vi "Equation.vi"(5 "Target height":dbl, 6 "Auto find":bool, 7 "Distance on ground (X)":dbl, 8 "RPM":dbl, 9 "zAvit":dbl) -> (0 "Risky!":bool, 1 "Calculated height":dbl, 2 "RPM":dbl, 3 "zAvit":dbl, 4 "Capable":bool)   [LabVIEW 2012]
panel:
  in  "K6":dbl
  in  "K5":dbl
  in  "K4":dbl
  in  "K3":dbl
  in  "K2":dbl
  in  "K1":dbl
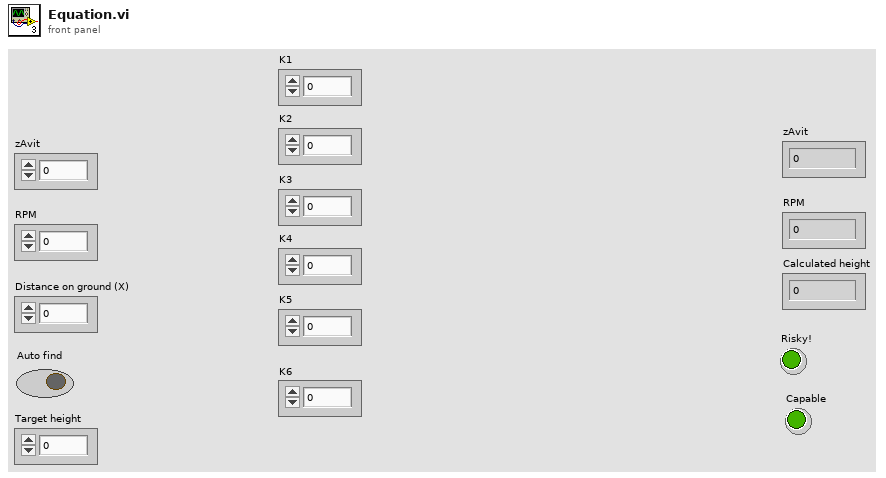
[diagram p1: front panel]
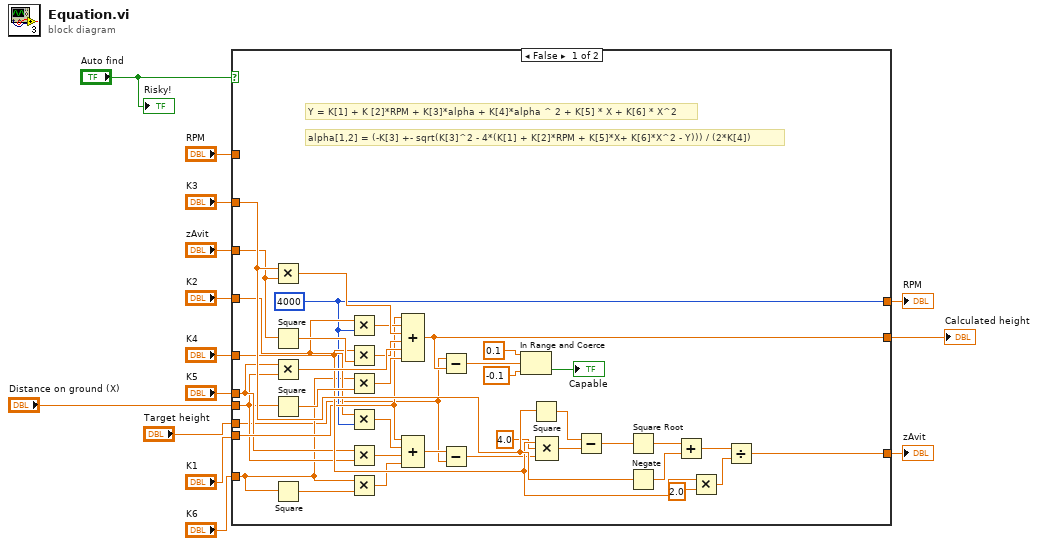
[diagram p0: block diagram]
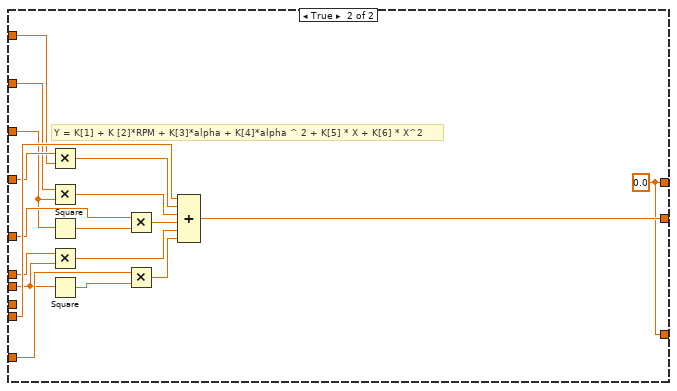
[diagram p2: hidden frame]
diagram:
  n1 = case shown="False" "Auto find" {
    tunnel: "K1" -> [w28 w65]
    tunnel: "K2" -> [w27 w64]
    tunnel: "RPM" -> [_ w63]
    tunnel: "K3" -> [w36 w62]
    tunnel: "K4" -> [w30 w61]
    tunnel: "zAvit" -> [w35 w56]
    tunnel: "K5" -> [w24 w59]
    tunnel: "K6" -> [w20 w58]
    tunnel: "Distance on ground (X)" -> [w23 w55]
    tunnel: [w26 w53] -> w4
    tunnel: [w33 w54] -> w3
    tunnel: [w47 w53] -> w2
    tunnel: "Target height" -> [w17 _]
    frame False {
      w26 = 4000
      # "alpha[1,2] = (-K[3] +- sqrt(K[3]^2 - 4*(K[1] + K[2]*RPM + K[5]*X+ K[6]*X^2 - Y))) / (2*K[4])"
      # "Y = K[1] + K [2]*RPM + K[3]*alpha + K[4]*alpha ^ 2 + K[5] * X + K[6] * X^2"
      n2 = Multiply(x=w36, y=w35) -> (x*y=w43:dbl)
      n3 = Square(x=w35) -> (x^2=w41:dbl)
      n4 = Multiply(x=w24, y=w23) -> (x*y=w45:dbl)
      n5 = Square(x=w23) -> (x^2=w34:dbl)
      n6 = Square(x=w20) -> (x^2=w21:dbl)
      n7 = Multiply(x=w27, y=w26) -> (x*y=w42:dbl)
      n8 = Multiply(x=w30, y=w41) -> (x*y=w44:dbl)
      n9 = Multiply(x=w20, y=w34) -> (x*y=w46:dbl)
      n10 = Multiply(x=w27, y=w26) -> (x*y=w25:dbl)
      n11 = Multiply(x=w24, y=w23) -> (x*y=w22:dbl)
      n12 = Multiply(x=w20, y=w21) -> (x*y=w18:dbl)
      n13 = Compound Arithmetic op=ADD(w28, w42, w43, w44, w45, w46) -> (w33:dbl)
      n14 = Compound Arithmetic op=ADD(w28, w25, w22, w18) -> (w19:dbl)
      n15 = Subtract(x=w17, y=w33) -> (x-y=w40:dbl)
      n16 = Subtract(x=w19, y=w17) -> (x-y=w16:dbl)
      n17 = In Range and Coerce(upper limit=0.1, x=w40, lower limit=-0.1) -> (In Range?=→"Capable":bool)  [unwired: 1 out]
      n18 = Square(x=w36) -> (x^2=w31:dbl)
      n19 = Compound Arithmetic op=MULTIPLY(w30, 4.0 ("y"), w16) -> (w15:dbl)
      n20 = Subtract(x=w31, y=w15) -> (x-y=w32:dbl)
      n21 = Square Root(x=w32) -> (sqrt(x)=w50:dbl)
      n22 = Negate(x=w36) -> (-x=w49:dbl)
      n23 = Add(x=w50, y=w49) -> (x+y=w48:dbl)
      n24 = Multiply(x=w30, y=2.0) -> (x*y=w51:dbl)
      n25 = Divide(x=w48, y=w51) -> (x/y=w47:dbl)
    }
    frame True {
      w53 = 0.0
      # "Y = K[1] + K [2]*RPM + K[3]*alpha + K[4]*alpha ^ 2 + K[5] * X + K[6] * X^2"
      n26 = Multiply(x=w64, y=w63) -> (x*y=w66:dbl)
      n27 = Multiply(x=w62, y=w56) -> (x*y=w67:dbl)
      n28 = Square(x=w56) -> (x^2=w60:dbl)
      n29 = Multiply(x=w59, y=w55) -> (x*y=w69:dbl)
      n30 = Square(x=w55) -> (x^2=w57:dbl)
      n31 = Multiply(x=w61, y=w60) -> (x*y=w68:dbl)
      n32 = Multiply(x=w58, y=w57) -> (x*y=w70:dbl)
      n33 = Compound Arithmetic op=ADD(w65, w66, w67, w68, w69, w70) -> (w54:dbl)
    }
  }
  "zAvit" <- w2
  "RPM" <- w4
  "Calculated height" <- w3
  "Risky!" <- "Auto find"
